vi "Error Check.vi"(8 "error in":errorcluster, 10 "Error Query Command":string, 11 "Device Details in":T1={"Device Port Number"=2001, "Device IP"="192.168.1.1.100", "Timeout"=5000, "Port Number"=1234, "Connection ID"=refnum}) -> (0 "error out":errorcluster, 3 "Device Details out":T1={"Device Port Number"=2001, "Device IP"="192.168.1.1.100", "Timeout"=5000, "Port Number"=1234, "Connection ID"=refnum})   [LabVIEW 2020, in "Plugin Instrument Driver.lvlib" / "UDP.lvclass"]
doc: "This VI Sets the error query command and reads the response from instrument."
uses:
  UDP.lvclass
  Typedefs/Device Details.ctl
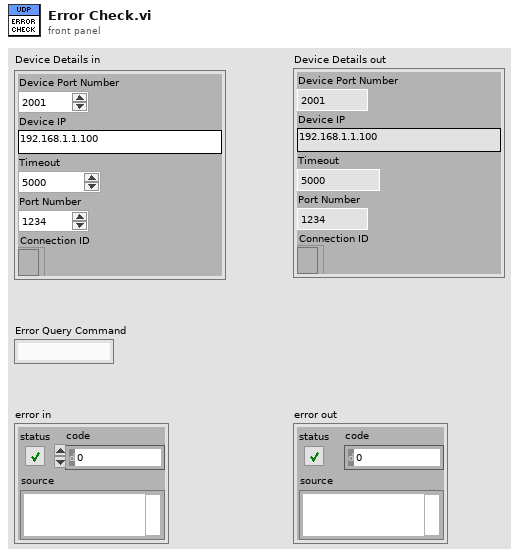
[diagram p1: front panel]
types:
  T1 = typedef "Plugin Instrument Driver.lvlib/UDP.lvclass/Device Details.ctl" = cluster{"Device Port Number":u16, "Device IP":string, "Timeout":i32, "Port Number":u16, "Connection ID":refnum<k16>}
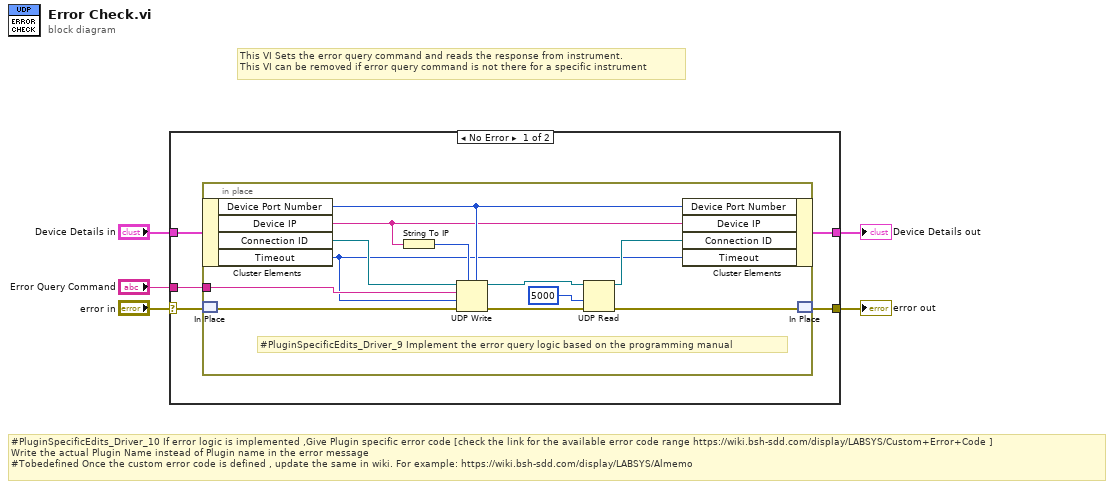
[diagram p0: block diagram]
diagram:
  # "This VI Sets the error query command and reads the response from instrument. \nThis VI can be removed if error query command is not there for a specific instrument"
  # "#PluginSpecificEdits_Driver_10 If error logic is implemented ,Give Plugin specific error code [check the link for the available error code range https://wiki.bsh-sdd.com/display/LABSYS/Custom+Error+Code ]\nWrite the actual Plugin Name instead of Plugin name in the error message\n#Tobedefined Once the custom error code is defined , update the same in wiki. For example: https://wiki.bsh-sdd.com/display/LABSYS/Almemo"
  n1 = case shown="No Error" "error in" {
    selector: "error in" -> [w9 w24]
    tunnel: [w7 w24] -> w5
    tunnel: "Device Details in" -> [w10 w23]
    tunnel: "Error Query Command" -> [w6 _]
    tunnel: [w8 w23] -> w1
    frame No Error {
      n2 = in-place {
        in-place-border: w6 -> [w14]
        # "#PluginSpecificEdits_Driver_9 Implement the error query logic based on the programming manual"
        n3 = in-place-cluster #1(w10) -> ("Device Port Number"=w13:u16, "Device IP"=w12:string, "Connection ID"=w17:refnum<k16>, "Timeout"=w11:i32)
        n4 = in-place-match #2(w9) -> (w18:errorcluster)
        n5 = String To IP(1:w12) -> (0:w20:u32)
        n6 = UDP Write(address=w20, port or service name=w13, connection ID=w17, data in=w14, 8:w18, 9:w11) -> (error out=w21:errorcluster, 3:w19:refnum<k16>)
        n7 = UDP Read(connection ID=w19, timeout ms (25000)=5000, 8:w21) -> (error out=w15:errorcluster, 3:w16:refnum<k16>)  [unwired: 1 in, 3 out]
        n8 = in-place-cluster #1("Device Port Number"=w13, "Device IP"=w12, "Connection ID"=w16, "Timeout"=w11) -> (w8:T1)
        n9 = in-place-match #2(w15) -> (w7:errorcluster)
      }
    }
    frame Error {
    }
  }
  "error out" <- w5
  "Device Details out" <- w1
